vi "NI 9230 pd-demodulation (Host).vi"() -> ()   [LabVIEW 2021]
doc: "This VI runs on the host device. The host can be a Windows PC or Real-Time target. The example reads a buffer of single point values from all three channels of the NI 9232."
uses:
  <vilib>/userDefined/High Color/nirio_resource_hc.ctl
  <vilib>/LabVIEW Targets/FPGA/cRIO/shared/nicrio_ModuleControls/nicrio_cRIO-9232_ConfigModeRing.ctl
  <vilib>/LabVIEW Targets/FPGA/cRIO/shared/nicrio_ModuleControls/nicrio_cRIO-9230_DataRatesRing2.ctl
  <vilib>/FPGAPlugInAG/cRIO-9053/niLvFpga_Open_cRIO-9053.vi
  <vilib>/rvi/interface/common/dynamic/niFpgaDynamicAddResources.vi
  <vilib>/FPGAPlugInAG/Dynamic/niLvFpga_Reset_Dynamic.vi
  <vilib>/Utility/error.llb/Error Cluster From Error Code.vi
  <vilib>/rvi/errors/niLvFpgaAdjustHostInterfaceError.vi
  <vilib>/FPGAPlugInAG/Dynamic/niLvFpga_Run_Dynamic.vi
  <vilib>/RVI Host/nirviSupport.llb/nirviErrorClusterFromErrorCode.vi
  <vilib>/LabVIEW Targets/FPGA/RIO/CompactRIO/cRIO-91xx/cRIO-91XX_ReadTEDSImpl.vi
  <vilib>/FPGAPlugInAG/Dynamic/niLvFpga_Close_Dynamic.vi
  <vilib>/Utility/file.llb/Write Delimited Spreadsheet (DBL).vi
  <vilib>/rvi/interface/nirviOpenFPGA/nirviOpenFPGA.xnode
  FPGA Bitfiles/ni9230gettingsta_FPGATarget2_NI9230GettingSta_c6zQ8chLpPs.lvbitx
  <vilib>/rvi/interface/nirviMethod/nirviMethod.xnode
  <vilib>/rvi/interface/nirviReadWriteControl/nirviReadWriteControl.xnode
  <vilib>/rvi/interface/nirviCloseFPGA/nirviCloseFPGA.xnode
  <vilib>/rvi/interface/Simulation/niFpgaSimulationCallBeginRW.vi
  <vilib>/rvi/interface/nirviMethod/StockFPGA_InlinedMethodWaitForSingleIRQ.vi
  <vilib>/FPGAPlugInAG/Dynamic/niLvFpga_WaitOnIrq_Dynamic.vi
  <vilib>/FPGAPlugInAG/Dynamic/niLvFpga_AcknowledgeIrq_Dynamic.vi
  <vilib>/FPGAPlugInAG/Dynamic/niLvFpga_ReadFifo_Dynamic.vi
  <vilib>/rvi/errors/niLvFpgaMergeErrorWithErrorCode.vi
  NiFpgaLv.dll
panel:
  out "Num pts Pos 2":i32=32
  out "Read FIFO loop time":u32=100
  out "Sample Rate":dbl=12800.0
  out "High level":bool=TRUE
  out "Low level":bool
  out "Demodulated Signal":dbl(graph)=0.4301605224609375
  out "Num pts Neg":i32=64
  out "Original Signal middle":dbl(graph)=0.4387359619140625
  out "middle point pos":dbl=0.4387359619140625
  out "Modulation frequency":dbl=100.0
  out "Num pts Pos":i32=64
  out "Queue":i32
  in  "Consumer loop update rate (ms)":u32=10
  out "Consumer loop time":u32=101
  out "XY Graph":cluster{dbl[], dbl[]}(graph)
  in  "Input Configuration 2":T1=1 items=["AC Coupled", "DC Coupled", "IEPE AC Coupled"]
  in  "Input Configuration 1":T1=1 items=["AC Coupled", "DC Coupled", "IEPE AC Coupled"]
  in  "Save data":bool caption="Enable"
  in  "Filename":path=path "C:/Users/data/2023_05_15_NI9230_pd-demodulation-12_8ks_100Hzmod_ch1_top_ch2_demod_001.lvm"
  in  "Host Loop update rate (ms)":u32=100
  in  "Data Rate":T2=10 items=["12.800 kS/s (NI 9230)"=10, "11.378 kS/s (NI 9230)"=36, "10.240 kS/s (NI 9230)"=21, "9.309 kS/s (NI 9230)"=44, "8.533 kS/s (NI 9230)"=14, "7.877 kS/s (NI 9230)"=52, "7.314 kS/s (NI 9230)"=29, "6.827 kS/s (NI 9230)"=60, "6.400 kS/s (NI 9230)"=18, "6.024 kS/s (NI 9230)"=68, "5.689 kS/s (NI 9230)"=37, "5.389 kS/s (NI 9230)"=76, "5.120 kS/s (NI 9230)"=22, "4.876 kS/s (NI 9230)"=84, "4.655 kS/s (NI 9230)"=45, "4.452 kS/s (NI 9230)"=92, "4.267 kS/s (NI 9230)"=26, "4.096 kS/s (NI 9230)"=100, "3.938 kS/s (NI 9230)"=53, "3.657 kS/s (NI 9230)"=30, "3.413 kS/s (NI 9230)"=61, "3.200 kS/s (NI 9230)"=34, "3.012 kS/s (NI 9230)"=69, "2.844 kS/s (NI 9230)"=38, "2.695 kS/s (NI 9230)"=77, "2.560 kS/s (NI 9230)"=42, "2.438 kS/s (NI 9230)"=85, "2.327 kS/s (NI 9230)"=46, "2.226 kS/s (NI 9230)"=93, "2.133 kS/s (NI 9230)"=50, "2.048 kS/s (NI 9230)"=101, "1.969 kS/s (NI 9230)"=54, "1.829 kS/s (NI 9230)"=58, "1.707 kS/s (NI 9230)"=62, "1.600 kS/s (NI 9230)"=66, "1.506 kS/s (NI 9230)"=70, "1.422 kS/s (NI 9230)"=74, "1.347 kS/s (NI 9230)"=78, "1.280 kS/s (NI 9230)"=82, "1.219 kS/s (NI 9230)"=86, "1.164 kS/s (NI 9230)"=90, "1.113 kS/s (NI 9230)"=94, "1.067 kS/s (NI 9230)"=98, "1.024 kS/s (NI 9230)"=102, "0.985 kS/s (NI 9230)"=106]
  in  "stop":bool
  out "Elements Remaining":u32
  out "FPGA error out":errorcluster
  out "Host error out":errorcluster
  out "Open Loop":bool[](array[boolean])
  out "Short Circuit":bool[](array[boolean])
  out "Data FIFO Full":bool
  in  "Input Configuration 0":T1=1 items=["AC Coupled", "DC Coupled", "IEPE AC Coupled"]
  in  "TEDS Template File Directory":path=path "C:/"
  in  "Display TEDS Data":bool
  in  "RIO Device":T3="RIO0"
  out "Waveform Graph":waveform(dbl)[](graph)=[{"t0"=timestamp(0 s since 1904-01-01), "dt"=7.8125e-05, "Y"=array[1284 elements]}, {"t0"=timestamp(0 s since 1904-01-01), "dt"=7.8125e-05, "Y"=array[1284 elements]}, {"t0"=timestamp(0 s since 1904-01-01), "dt"=7.8125e-05, "Y"=array[1284 elements]}]
  # "Overview: Demonstrates how to acquire data from the NI 9230\nRequirements: LabVIEW Full Development System, LV FPGA, and NI RIO\nInstructions: \n1. Run this VI."
  # "Resource Parameters"
  # "Timing Parameters"
  # "Ch0"
  # "Ch1"
  # "Ch2"
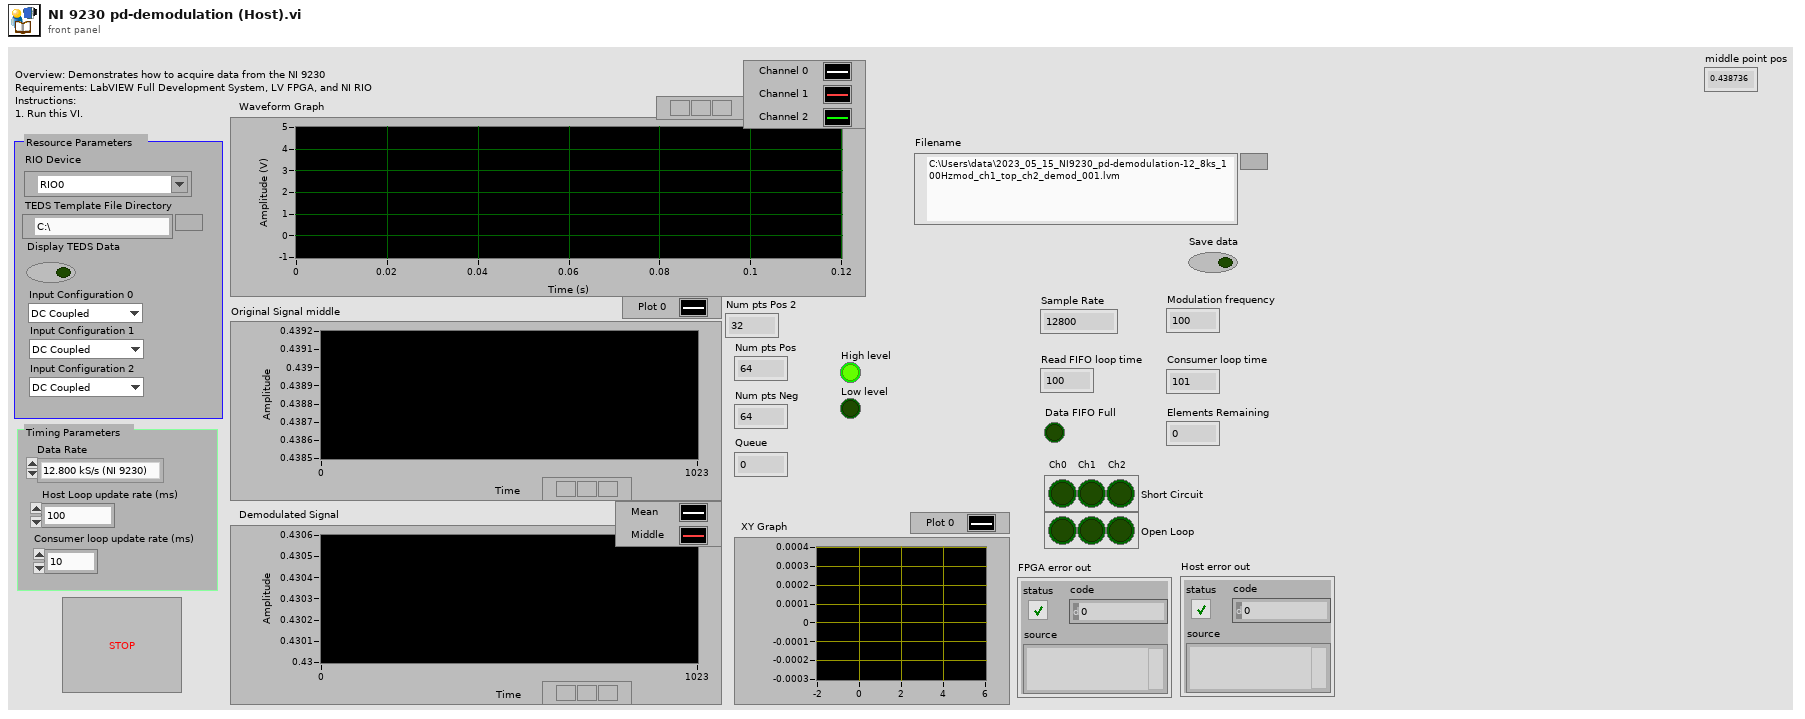
[diagram p1: front panel]
types:
  T1 = typedef "nicrio_cRIO-9232_ConfigModeRing.ctl" = u8
  T2 = typedef "nicrio_cRIO-9230_DataRatesRing2.ctl" = u8
  T3 = typedef "nirio_resource_hc.ctl" = tag
  T4 = cluster{"TEDS Error?":bool, "TEDS Error":string, "TEDS Data":string[][]}
  T5 = cluster{"output waveform 2":waveform(dbl), "output waveform 3":waveform(dbl)}
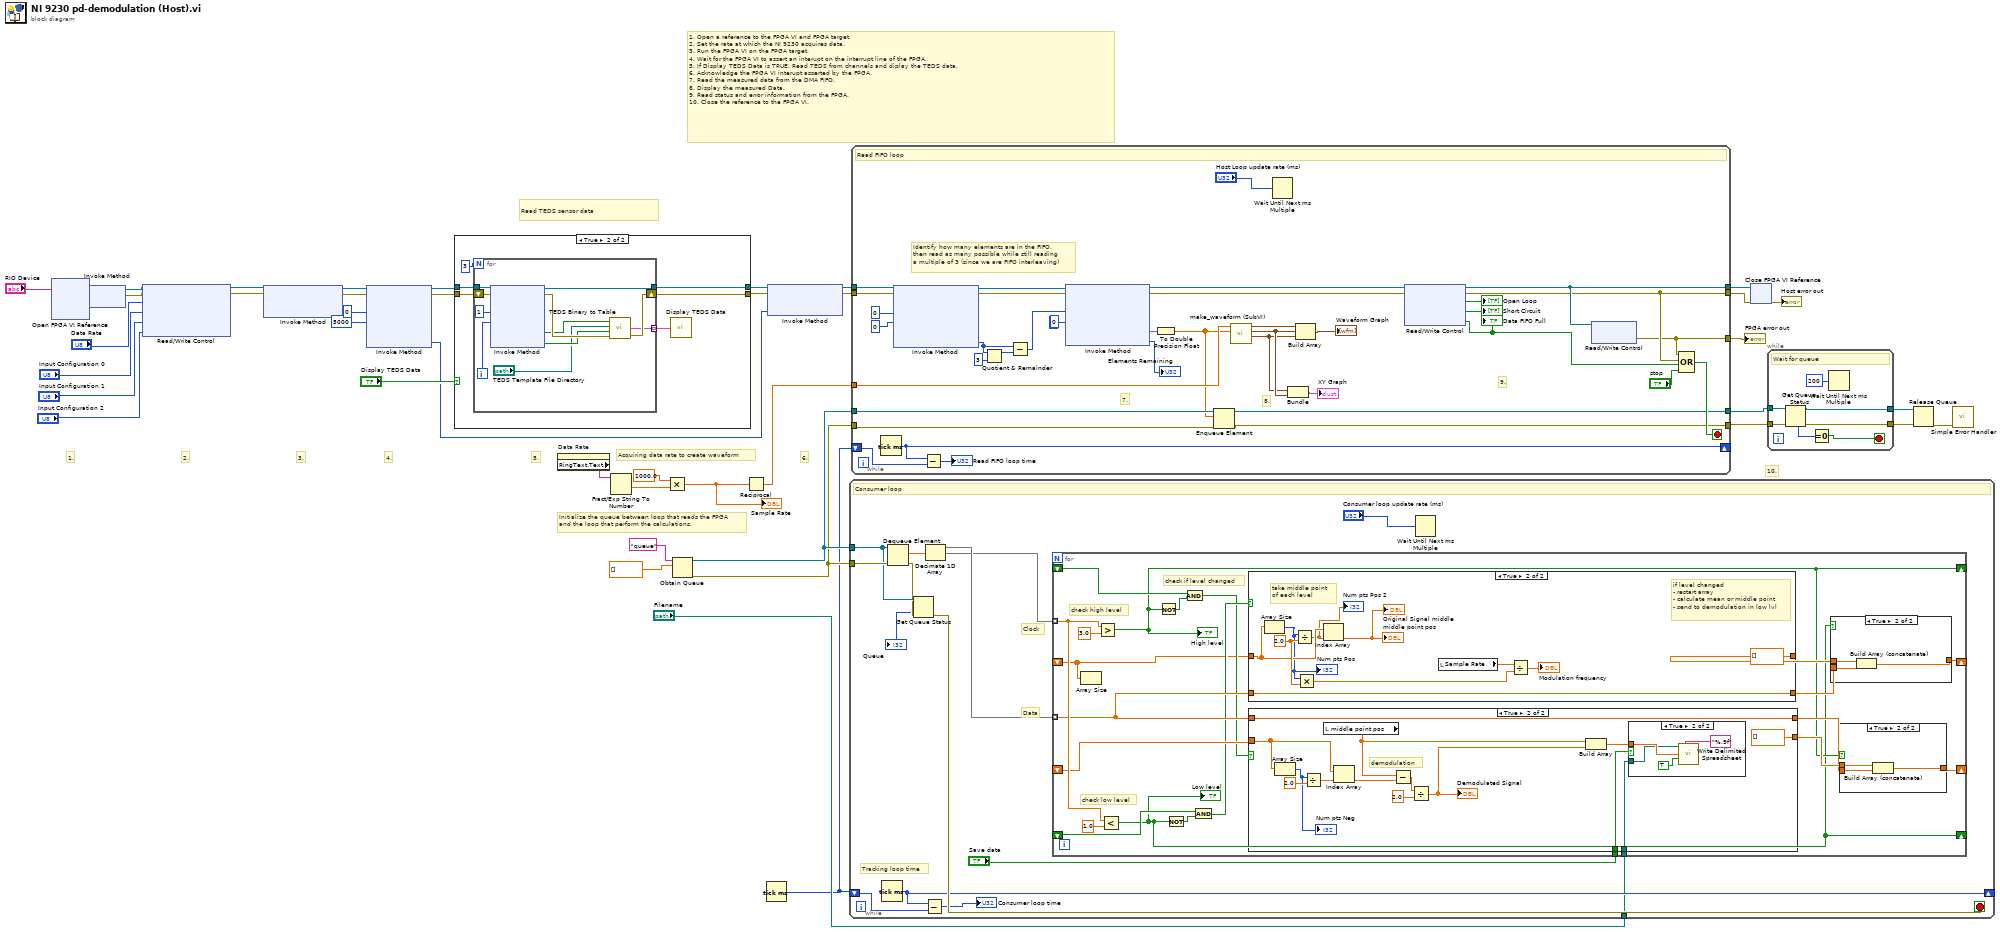
[diagram p0: block diagram]
diagram:
  # "Initialize the queue between loop that reads the FPGA\nand the loop that perform the calculations."
  # "Acquiring data rate to create waveform"
  # "10."
  # "6."
  # "5."
  # "3."
  # "4."
  # "2."
  # "1."
  # "1. Open a reference to the FPGA VI and FPGA target.\n2. Set the rate at which the NI 9230 acquires data.  \n3. Run the FPGA VI on the FPGA target. \n4. Wait for the FPGA VI to assert an interupt on the interrupt line of the FPGA.\n5. If Display TEDS Data is TRUE, Read TEDS from channels and diplay the TEDS data.\n6. Acknowledge the FPGA VI interupt asserted by the FPGA.\n7. Read the measured data from the DMA FIFO.\n8. Display the measured Data.\n9. Read status and error information from the FPGA.\n10. Close the reference to the FPGA VI."
  # "Read TEDS sensor data"
  n1 = xnode "Open FPGA VI Reference"("resource name"="RIO Device") -> ("FPGA VI Reference Out"=w23:refnum<k20>, "error out"=w31:errorcluster)  [unwired: 1 in]
  n2 = xnode "Invoke Method"("FPGA VI Reference In"=w23, "error in"=w31) -> ("FPGA VI Reference Out"=w22:refnum<k20>, "error out"=w24:errorcluster)
  n3 = xnode "Read/Write Control"("FPGA VI Reference In"=w22, "error in"=w24, "Data Rate"="Data Rate", "Input Configuration 0"="Input Configuration 0", "Input Configuration 1"="Input Configuration 1", "Input Configuration 2"="Input Configuration 2") -> ("FPGA VI Reference Out"=w35:refnum<k20>, "error out"=w34:errorcluster)
  n4 = xnode "Invoke Method"("FPGA VI Reference In"=w35, "error in"=w34) -> ("FPGA VI Reference Out"=w33:refnum<k20>, "error out"=w32:errorcluster)  [unwired: 1 in]
  n5 = xnode "Invoke Method"("FPGA VI Reference In"=w33, "error in"=w32, "IRQ Number(s)"=0, "Timeout (ms)"=5000 ("Timeout")) -> ("FPGA VI Reference Out"=w40:refnum<k20>, "error out"=w39:errorcluster, "IRQ(s) Asserted"=w36:i32)  [unwired: 1 out]
  n6 = case shown="True" "Display TEDS Data" {
    tunnel: w40 -> [w45 w51]
    tunnel: [w45 w50] -> w38
    tunnel: w39 -> [w44 w49]
    tunnel: [w44 w46] -> w37
    frame False {
    }
    frame True {
      n7 = for {
        N: 3 -> [_]
        tunnel: w51 -> [w62]
        tunnel: [w61] -> w50
        tunnel: [w56] -> w47 mode=indexing
        shift-right: [w57] -> w46
        shift-left: w49 -> [w60]
        i -> [w55]
        n8 = xnode "Invoke Method"("FPGA VI Reference In"=w62, "error in"=w60, "Slot"=1, "Channel"=w55) -> ("FPGA VI Reference Out"=w61:refnum<k20>, "error out"=w58:errorcluster, "TEDS Binary"=w53:bool[], "v0.9 (TEDS)"=w54:bool)
        n9 = call "TEDS Binary to Table.vi"("error in"=w58, "v0.9 TEDS (F)"=w54, "template file directory"="TEDS Template File Directory", "TEDS Binary"=w53) -> ("error out"=w57:errorcluster, "TEDS"=w56:T4)  [unwired: 1 out]
      }
      n10 = call "Display TEDS Data.vi"("TEDS Array"=w47) -> ()  [unwired: 4 out]
    }
  }
  n11 = property on="Data Rate" class="Ring (strict)"() -> ("RingText.Text"=w13:string)  [unwired: 2 in, 2 out]
  n12 = Fract/Exp String To Number(string=w13) -> (number=w16:dbl)  [unwired: 4 out]
  n13 = Multiply(x=1000.0, y=w16) -> (x*y=w1:dbl)
  "Sample Rate" <- w1
  n14 = Obtain Queue(name (unnamed)="queue", element data type=dbl[] []) -> (queue out=w5:refnum<queue>, error out=w4:errorcluster)  [unwired: 3 in, 1 out]
  n15 = Reciprocal(x=w1) -> (1/x=w14:dbl)
  n16 = Tick Count (ms)() -> (millisecond timer value=w2:u32)
  n17 = xnode "Invoke Method"("FPGA VI Reference In"=w38, "error in"=w37, "IRQ Number(s)"=w36) -> ("FPGA VI Reference Out"=w28:refnum<k20>, "error out"=w27:errorcluster)
  n18 = while {
    tunnel: w5 -> [w74]
    tunnel: w4 -> [w76]
    shift-right: [w68] -> _
    shift-left: w2 -> [w67]
    tunnel: "Filename" -> [w65]
    stop <- w72 stop-if-true
    # "Tracking loop time"
    # "Data"
    # "Clock"
    # "Consumer loop"
    n19 = Tick Count (ms)() -> (millisecond timer value=w68:u32)
    n20 = Dequeue Element(queue=w74, error in (no error)=w76) -> (element=w64:dbl[], error out=w73:errorcluster)  [unwired: 1 in, 2 out]
    n21 = Get Queue Status(queue=w74, error in (no error)=w73) -> (error out=w72:errorcluster, # elements in queue=→"Queue":i32)  [unwired: 1 in, 6 out]
    n22 = Subtract(x=w68, y=w67) -> (x-y=→"Consumer loop time":u32)
    n23 = Decimate 1D Array(w64) -> (w75:dbl[], w70:dbl[])  [unwired: 1 out]
    n24 = for {
      tunnel: w70 -> [w93] mode=indexing
      shift-right: [w82] -> _
      shift-left: _ -> [w92]
      shift-right: [w81] -> _
      shift-left: _ -> [w94]
      shift-right: [w89] -> _
      shift-left: _ -> [w91]
      shift-right: [w90] -> _
      shift-left: _ -> [w77]
      tunnel: w75 -> [w84] mode=indexing
      tunnel: "Save data" -> [w79]
      tunnel: w65 -> [w78]
      # "check low level"
      # "check high level"
      # "check if level changed"
      n25 = Array Size(array=w77) -> ()  [unwired: 1 out]
      n26 = Greater?(x=w93, y=3.0) -> (0:w82:bool)
      "High level" <- w82
      n27 = Less?(x=w93, y=1.0) -> (x < y?=w81:bool)
      "Low level" <- w81
      n28 = Not(x=w82) -> (.not. x?=w97:bool)
      n29 = Not(x=w81) -> (.not. x?=w95:bool)
      n30 = And(x=w92, y=w97) -> (x .and. y?=w80:bool)
      n31 = And(x=w94, y=w95) -> (x .and. y?=w83:bool)
      n32 = case shown="True" w83 {
        tunnel: [w100 dbl[] []] -> w87
        tunnel: w77 -> [w100 w104]
        tunnel: [w99 w110] -> w86
        tunnel: w84 -> [w99 w110]
        frame False {
        }
        frame True {
          w108 = 2.0 ("y")
          # "if level changed\n- restart array\n- calculate mean or middle point\n- send to demodulation in low lvl"
          # "take middle point \nof each level"
          n33 = Array Size(array=w104) -> (size(s)=w103:i32)
          "Num pts Pos" <- w103
          n34 = Divide(x=w103, y=w108) -> (x/y=w101:dbl)
          "Num pts Pos 2" <- w101
          n35 = Multiply(x=w103, y=w108) -> (x*y=w106:dbl)
          n36 = Index Array(array=w104, index=w101) -> (element=→"Original Signal middle" →"middle point pos":dbl)
          n37 = local read "Sample Rate"() -> (w107:dbl)
          n38 = Divide(x=w107, y=w106) -> (x/y=→"Modulation frequency":dbl)
        }
      }
      n39 = case shown="True" w80 {
        tunnel: [w112 dbl[] []] -> w88
        tunnel: w91 -> [w112 w115]
        tunnel: [w111 w126] -> w85
        tunnel: w84 -> [w111 w126]
        tunnel: w79 -> [_ w120]
        tunnel: w78 -> [_ w118]
        frame False {
        }
        frame True {
          # "demodulation"
          n40 = Array Size(array=w115) -> (size(s)=w117:i32)
          "Num pts Neg" <- w117
          n41 = Divide(x=w117, y=2.0) -> (x/y=w116:dbl)
          n42 = local read "middle point pos"() -> (w113:dbl)
          n43 = Index Array(array=w115, index=w116) -> (element=w122:dbl)
          n44 = Subtract(x=w113, y=w122) -> (x-y=w124:dbl)
          n45 = Divide(x=w124, y=2.0) -> (x/y=w114:dbl)
          "Demodulated Signal" <- w114
          n46 = Build Array(w113, w114) -> (w119:dbl[])
          n47 = case shown="True" w120 {
            tunnel: w119 -> [_ w129]
            tunnel: w118 -> [_ w128]
            frame False {
            }
            frame True {
              n48 = call-poly <vilib>:"Write Delimited Spreadsheet.vi"("file path (dialog if empty)"=w128, "format (%.3f)"="%.9f", "1D data"=w129, "append to file? (new file:F)"=TRUE) -> ()  [unwired: 10 in, 2 out]
            }
          }
        }
      }
      n49 = case shown="True" w81 {
        tunnel: w87 -> [w135 w138]
        tunnel: [w135 w136] -> w90
        tunnel: w86 -> [_ w137]
        frame False {
        }
        frame True {
          n50 = Build Array (concatenate)(w138, w137) -> (w136:dbl[])
        }
      }
      n51 = case shown="True" w82 {
        tunnel: w88 -> [w131 w134]
        tunnel: w85 -> [_ w133]
        tunnel: [w131 w132] -> w89
        frame False {
        }
        frame True {
          n52 = Build Array (concatenate)(w134, w133) -> (w132:dbl[])
        }
      }
    }
    n53 = Wait Until Next ms Multiple(millisecond multiple="Consumer loop update rate (ms)") -> ()  [unwired: 1 out]
  }
  n54 = while {
    tunnel: [w166] -> w25
    tunnel: [w165] -> w30
    tunnel: w28 -> [w156]
    tunnel: w27 -> [w155]
    tunnel: [w164] -> w21
    tunnel: w14 -> [w151]
    tunnel: w5 -> [w150]
    tunnel: w4 -> [w148]
    tunnel: [w147] -> w7
    tunnel: [w146] -> w6
    shift-right: [w140] -> _
    shift-left: w2 -> [w141]
    stop <- w176 stop-if-true
    (unwired) 0 ("Timeout (ms)")
    # "7."
    # "8."
    # "9."
    # "Identify how many elements are in the FIFO, \nthen read as many possible while still reading\na multiple of 3 (since we are FIFO interleaving)"
    # "Read FIFO loop"
    n55 = Tick Count (ms)() -> (millisecond timer value=w140:u32)
    n56 = xnode "Invoke Method"("FPGA VI Reference In"=w156, "error in"=w155, "Number of Elements"=u32 0, "Timeout (ms)"=0) -> ("FPGA VI Reference Out"=w158:refnum<k20>, "error out"=w157:errorcluster, "Elements Remaining"=w163:u32)  [unwired: 1 out]
    n57 = Subtract(x=w140, y=w141) -> (x-y=→"Read FIFO loop time":u32)
    n58 = Quotient & Remainder(x=w163, y=u32 3) -> (x-y*floor(x/y)=w162:u32)  [unwired: 1 out]
    n59 = Subtract(x=w163, y=w162) -> (x-y=w159:u32)
    n60 = xnode "Invoke Method"("FPGA VI Reference In"=w158, "error in"=w157, "Number of Elements"=w159, "Timeout (ms)"=0 ("Timeout")) -> ("FPGA VI Reference Out"=w175:refnum<k20>, "error out"=w174:errorcluster, "Data"=w172:fxp<+/-,24,7>[], "Elements Remaining"=→"Elements Remaining":u32)
    n61 = To Double Precision Float(number=w172) -> (double precision float=w149:dbl[])
    n62 = Enqueue Element(queue=w150, element=w149, error in (no error)=w148) -> (queue out=w147:refnum<queue>, error out=w146:errorcluster)  [unwired: 1 in, 1 out]
    n63 = call "make_waveform (SubVI).vi"("Array"=w149, "Numeric"=w151) -> ("output waveform 2"=w142:waveform(dbl), "output waveform 3"=w143:waveform(dbl), "output waveform"=w144:waveform(dbl))  [unwired: 7 in]
    n64 = Wait Until Next ms Multiple(millisecond multiple="Host Loop update rate (ms)") -> ()  [unwired: 1 out]
    n65 = Bundle("output waveform 2"=w142, "output waveform 3"=w143) -> (→"XY Graph":T5)  [unwired: 1 in]
    n66 = Build Array(w144, w143, w142) -> (→"Waveform Graph":waveform(dbl)[])
    n67 = xnode "Read/Write Control"("FPGA VI Reference In"=w175, "error in"=w174) -> ("FPGA VI Reference Out"=w166:refnum<k20>, "error out"=w165:errorcluster, "Open Loop"=→"Open Loop":bool[], "Short Circuit"=→"Short Circuit":bool[], "Data FIFO Full"=w169:bool)
    "Data FIFO Full" <- w169
    n68 = xnode "Read/Write Control"("FPGA VI Reference In"=w166) -> ("Error Out"=w164:errorcluster)  [unwired: 1 in, 2 out]
    n69 = Compound Arithmetic op=OR(w164, w165, w169, "stop") -> (w176:bool)
  }
  "FPGA error out" <- w21
  n70 = xnode "Close FPGA VI Reference"("FPGA VI Reference In"=w25, "error in"=w30) -> ("error out"=→"Host error out":errorcluster)
  n71 = while {
    tunnel: w7 -> [w183]
    tunnel: [w179] -> w10
    tunnel: w6 -> [w178]
    tunnel: [w177] -> w9
    stop <- w181 stop-if-true
    # "Wait for queue"
    n72 = Get Queue Status(queue=w183, error in (no error)=w178) -> (queue out=w179:refnum<queue>, error out=w177:errorcluster, # elements in queue=w182:i32)  [unwired: 1 in, 5 out]
    n73 = Equal To 0?(x=w182) -> (x = 0?=w181:bool)
    n74 = Wait Until Next ms Multiple(millisecond multiple=u32 200) -> ()  [unwired: 1 out]
  }
  n75 = Release Queue(queue=w10, error in (no error)=w9) -> (error out=w8:errorcluster)  [unwired: 1 in, 2 out]
  n76 = call <vilib>:"Simple Error Handler.vi"("error in (no error)"=w8) -> ()  [unwired: 4 in, 5 out]
